vi "get Test Component Directory.vi"() -> (3 "test component directory":path)   [LabVIEW 2017, in "Framework Property Tests.lvclass"]
uses:
  Framework Property Tests.lvclass
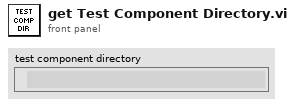
[diagram p1: front panel]
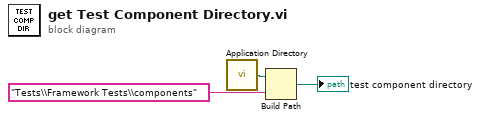
[diagram p0: block diagram]
diagram:
  n1 = call <vilib>:"Application Directory.vi"() -> ("Application Directory"=w1:path)
  n2 = Build Path(base path=w1, name or relative path="Tests\\Framework Tests\\components") -> (appended path=→"test component directory":path)
